vi "TGT_Query.vi"(0 "System no.":i32=1 min=1 max=4 step=1, 5 "error in":errorcluster) -> (14 "Timing":i32=1 min=1 step=1, 19 "error out":errorcluster)   [LabVIEW 2020]
doc: "Get trajectory timing. For further details, see Trajectories for Motion Paths in the controller user manual.\n\nC-867, C-884:"
panel:
  # "Get trajectory timing."
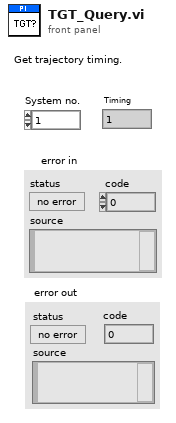
[diagram p1: front panel]
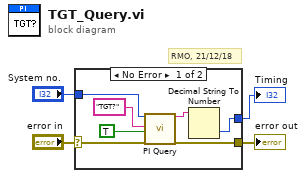
[diagram p0: block diagram]
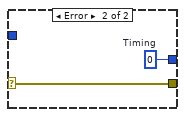
[diagram p2: hidden frame]
diagram:
  # "RMO, 21/12/18"
  n1 = case shown="No Error" "error in" {
    selector: "error in" -> [w5 w12]
    tunnel: [w7 w12] -> w4
    tunnel: "System no." -> [w9 _]
    tunnel: [w8 w13] -> w2
    frame No Error {
      n2 = call "PI Query.vi"("System no."=w9, "String to send"="TGT?", "Attach termination char.?"=TRUE ("Attach Linefeed?"), "error in"=w5) -> ("String read"=w6:string, "error out"=w7:errorcluster)  [unwired: 3 in, 11 out]
      n3 = Decimal String To Number(string=w6) -> (number=w8:i32)  [unwired: 3 out]
    }
    frame Error {
      w13 = 0  # Timing
    }
  }
  "error out" <- w4
  "Timing" <- w2
